vi "Bytes at port more than X.vi"(0 "X":u32, 2 "error IO":errorcluster, 3 "port in":refnum<visa-resource-name>) -> (6 "port out":refnum<visa-resource-name>, 7 "Bytes at port > X":bool, 9 "error out":errorcluster)   [LabVIEW 2013]
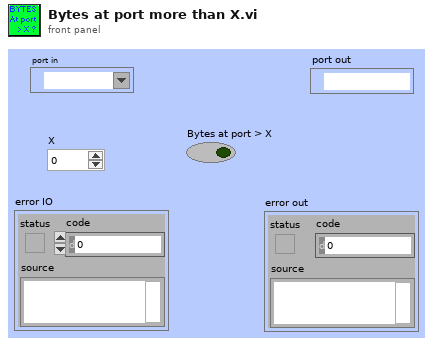
[diagram p1: front panel]
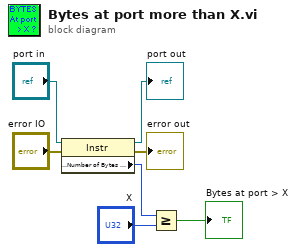
[diagram p0: block diagram]
diagram:
  n1 = property class="Instr"(reference="port in", error in="error IO") -> (reference out=→"port out":refnum<visa-resource-name>, error out=→"error out":errorcluster, "Serial Settings:Number of Bytes at Serial Port"=w2:u32)
  n2 = Greater Or Equal?(x=w2, y="X") -> (x >= y?=→"Bytes at port > X":bool)
